vi "WT300 Get Frequency.vi"(8 "error in (no error)":errorcluster, 10 "Update Rate (500m s)":dbl(ring)=0.5 format="%#_2f" items=["100m"=0.1, "250m"=0.25, "500m"=0.5, "1"=1.0, "2"=2.0, "5"=5.0], 11 "VISA Refnum in":refnum<visa-resource-name>) -> (0 "error out":errorcluster, 1 "Function":string[](array[string]), 2 "Measurement":dbl[](array[numeric]), 3 "VISA resource name out":refnum<visa-resource-name>)   [LabVIEW 2019]
uses:
  Public/Utility/Function/Create Function String (Frequency).vi
  Public/Data/Read Measurement (Normal).vi
  Yokogawa WT300 Series.lvlib
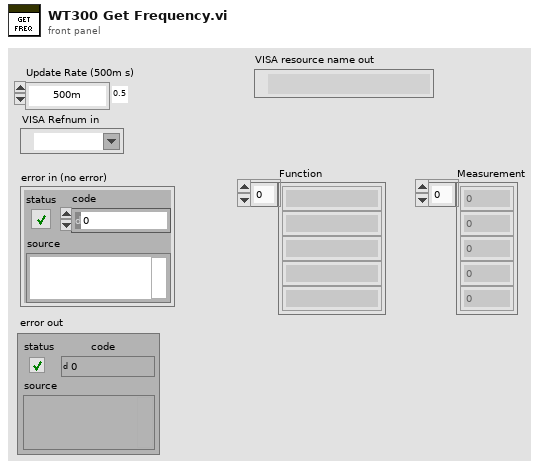
[diagram p1: front panel]
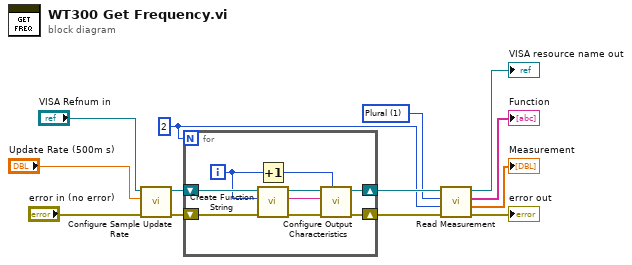
[diagram p0: block diagram]
diagram:
  w6 = 2
  w9 = 1 items=["One", "Plural"] ("Measure Item (1: Plural)")
  n1 = call "Configure Sample Update Rate.vi"("error in (no error)"="error in (no error)", "Update Rate (500m s)"="Update Rate (500m s)", "VISA resource name"="VISA Refnum in") -> ("error out"=w1:errorcluster, "VISA resource name out"=w2:refnum<visa-resource-name>)  [unwired: 7 in]
  n2 = for {
    N: w6 -> [_]
    shift-right: [w16] -> w10
    shift-left: w2 -> [w19]
    shift-right: [w17] -> w11
    shift-left: w1 -> [w18]
    i -> [w15]
    n3 = Increment(x=w15) -> (x+1=w14:i32)
    n4 = call-poly "Create Function String.vi"("error in (no error)"=w18, "Function (0: Frequency U)"=w15, "VISA resource name"=w19) -> ("error out"=w22:errorcluster, "Function String"=w21:string, "VISA resource name out"=w20:refnum<visa-resource-name>)  [unwired: 6 in]
    n5 = call "Configure Output Characteristics.vi"("Item (1)"=w14, "error in (no error)"=w22, "Function (Empty)"=w21, "VISA resource name"=w20) -> ("error out"=w17:errorcluster, "VISA resource name out"=w16:refnum<visa-resource-name>)  [unwired: 6 in]
  }
  n6 = call-poly "Read Measurement.vi"("error in (no error)"=w11, "Number of Item (15)"=w6, "Measure Item (1: Plural)"=w9, "VISA resource name"=w10) -> ("error out"=→"error out":errorcluster, "Measurement"=→"Measurement":dbl[], "Function"=→"Function":string[], "VISA resource name out"=→"VISA resource name out":refnum<visa-resource-name>)  [unwired: 4 in]
